vi "UDP.vi"() -> ()   [LabVIEW 2024]
panel:
  in  "stop":bool
  out "x = y?":bool
  out "error out 2":errorcluster
  out "error out":errorcluster
  in  "length (rest) 2":i32=3
  in  "offset (0) 2":i32=5
  out "substring 2":string
  out "data out 2":string
  in  "length (rest)":i32=3
  in  "offset (0)":i32=5
  out "substring":string
  out "data out":string
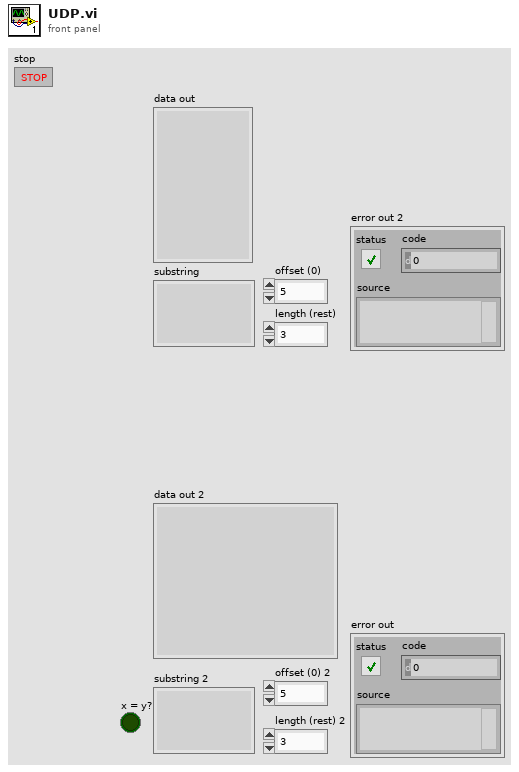
[diagram p1: front panel]
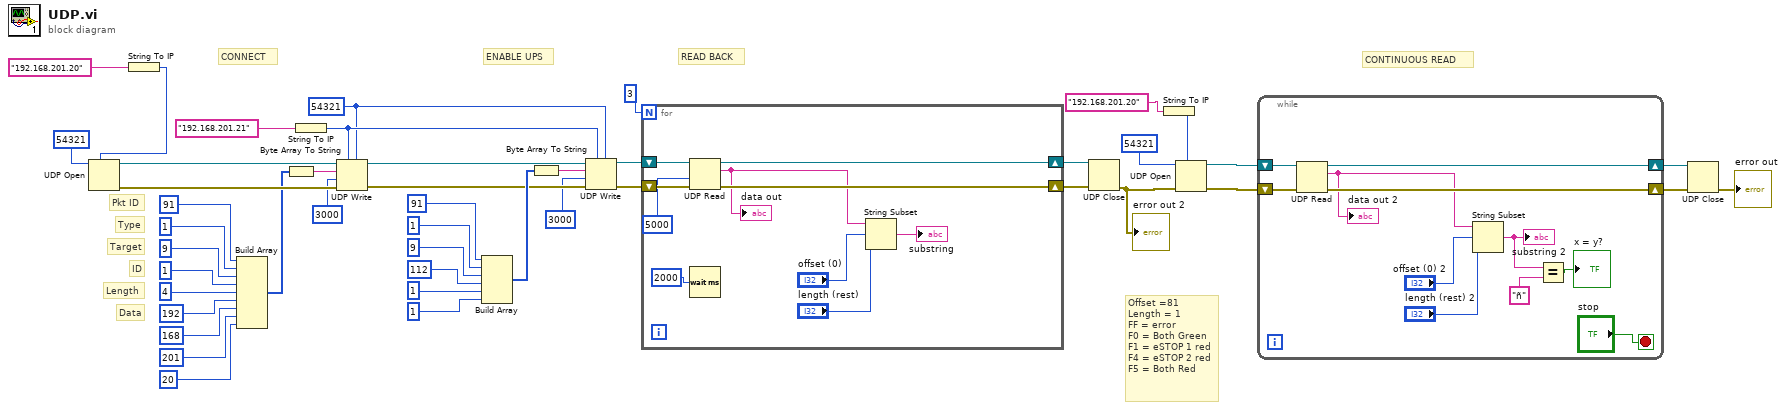
[diagram p0: block diagram]
diagram:
  w19 = u16 54321 ("port or service name")
  # "CONTINUOUS READ"
  # "Offset =81 \nLength = 1\nFF = error\nF0 = Both Green\nF1 = eSTOP 1 red\nF4 = eSTOP 2 red\nF5 = Both Red"
  # "Data"
  # "Length"
  # "ID"
  # "Target"
  # "Type"
  # "Pkt ID"
  # "READ BACK"
  # "ENABLE UPS"
  # "CONNECT"
  n1 = String To IP(1:"192.168.201.20" ("name")) -> (0:w10:u32)
  n2 = UDP Open(7:w10, 11:u16 54321 ("port")) -> (port=w43:refnum<k16>, 0:w44:errorcluster)  [unwired: 3 in, 1 out]
  n3 = Build Array(u8 91 ("element"), u8 1 ("element"), u8 9 ("element"), u8 1 ("element"), u8 4 ("element"), u8 192 ("element"), u8 168 ("element"), u8 201 ("element"), u8 20 ("element")) -> (w40:u8[])
  n4 = Byte Array To String(unsigned byte array=w40) -> (string=w41:string)
  n5 = String To IP(1:"192.168.201.21" ("name")) -> (0:w20:u32)
  n6 = UDP Write(address=w20, port or service name=w19, connection ID=w43, data in=w41, 8:w44, 9:3000 ("timeout ms (25000)")) -> (error out=w23:errorcluster, 3:w22:refnum<k16>)
  n7 = Build Array(u8 91 ("element"), u8 1 ("element"), u8 9 ("element"), u8 112 ("element"), u8 1 ("element"), u8 1 ("element")) -> (w29:u8[])
  n8 = Byte Array To String(unsigned byte array=w29) -> (string=w21:string)
  n9 = UDP Write(address=w20, port or service name=w19, connection ID=w22, data in=w21, 8:w23, 9:3000 ("timeout ms (25000)")) -> (error out=w14:errorcluster, 3:w15:refnum<k16>)
  n10 = for {
    N: 3 -> [_]
    shift-right: [w55] -> w17
    shift-left: w15 -> [w53]
    shift-right: [w54] -> w16
    shift-left: w14 -> [w52]
    n11 = UDP Read(connection ID=w53, timeout ms (25000)=5000, 8:w52) -> (data out=w51:string, error out=w54:errorcluster, 3:w55:refnum<k16>)  [unwired: 1 in, 2 out]
    "data out" <- w51
    n12 = Wait (ms)(milliseconds to wait=u32 2000) -> ()  [unwired: 1 out]
    n13 = String Subset(string=w51, offset (0)="offset (0)", length (rest)="length (rest)") -> (substring=→"substring":string)
  }
  n14 = UDP Close(connection ID=w17, 8:w16) -> (error out=w12:errorcluster)  [unwired: 1 out]
  "error out 2" <- w12
  n15 = String To IP(1:"192.168.201.20" ("name")) -> (0:w5:u32)
  n16 = UDP Open(7:w5, 8:w12, 11:u16 54321 ("port")) -> (port=w2:refnum<k16>, 0:w6:errorcluster)  [unwired: 2 in, 1 out]
  n17 = while {
    shift-right: [w66] -> w9
    shift-left: w6 -> [w61]
    shift-right: [w65] -> w8
    shift-left: w2 -> [w60]
    stop <- "stop" stop-if-true
    n18 = UDP Read(connection ID=w60, 8:w61) -> (data out=w64:string, error out=w66:errorcluster, 3:w65:refnum<k16>)  [unwired: 2 in, 2 out]
    "data out 2" <- w64
    n19 = String Subset(string=w64, offset (0)="offset (0) 2", length (rest)="length (rest) 2") -> (substring=w59:string)
    "substring 2" <- w59
    n20 = Equal?(x=w59, y="ñ") -> (x = y?=→"x = y?":bool)
  }
  n21 = UDP Close(connection ID=w8, 8:w9) -> (error out=→"error out":errorcluster)  [unwired: 1 out]
